vi "Destroy.vi"(8 "error in (no error)":errorcluster, 11 "Event Registration Refnum":refnum<event-registration>) -> (0 "error out":errorcluster)   [LabVIEW 2017, in "WebServiceImporter.lvlib" / "Main Panel.lvlib" / "Progress.lvlib" / "Events.lvlib"]
uses:
  <vilib>/Platform/WebService/Main Panel/Pages/Progress/Events/Events.lvlib
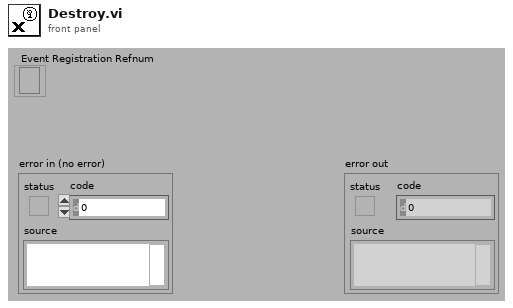
[diagram p1: front panel]
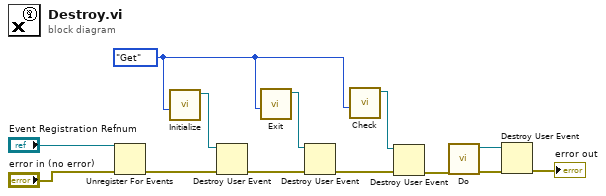
[diagram p0: block diagram]
diagram:
  w12 = enum16{"Get", "Set"}."Get" ("Operation")
  n1 = Unregister For Events(event registration refnum="Event Registration Refnum", error in="error in (no error)") -> (error out=w11:errorcluster)
  n2 = call <vilib>:"Initialize.vi"("Operation"=w12) -> ("user event (out)"=w10:refnum<user-event>)  [unwired: 10 in]
  n3 = Destroy User Event(user event=w10, error in=w11) -> (error out=w9:errorcluster)
  n4 = call <vilib>:"Exit.vi"("Operation"=w12) -> ("user event (out)"=w8:refnum<user-event>)  [unwired: 9 in, 1 out]
  n5 = Destroy User Event(user event=w8, error in=w9) -> (error out=w7:errorcluster)
  n6 = call <vilib>:"Check.vi"("Operation"=w12) -> ("user event (out)"=w6:refnum<user-event>)  [unwired: 10 in]
  n7 = Destroy User Event(user event=w6, error in=w7) -> (error out=w4:errorcluster)
  n8 = call <vilib>:"Do.vi"("error in (no error)"=w4) -> ("error out"=w3:errorcluster, "user event (out)"=w1:refnum<user-event>)  [unwired: 9 in]
  n9 = Destroy User Event(user event=w1, error in=w3) -> (error out=→"error out":errorcluster)
